vi "Lex Text-Inverted Section-Text.vi"(8 "Error In":errorcluster) -> (0 "Error Out":errorcluster)   [LabVIEW 2018, in "Tests.lvlib" / "Lexer.lvlib"]
uses:
  Lexer.lvlib
  src/Toolkit/Low-Level/Tokens/Text/Text.lvclass
  src/Toolkit/Low-Level/Tokens/InvertedSection/InvertedSection.lvclass
  src/Toolkit/Low-Level/Tokens/Keyable/Keyable.lvclass/Keyable.ctl
  src/Toolkit/Low-Level/Tokens/Keyable/Read Key.vi
  src/Toolkit/Low-Level/Support/Lex String.vi
  <vilib>/Utility/LVClass/Get LV Class Name.vi
  src/Toolkit/Low-Level/Tokens/Contentable/Contentable.lvclass
  src/Toolkit/Low-Level/Tokens/Keyable/Keyable.lvclass
  <vilib>/addons/_JKI Toolkits/Caraya/classes/Test/Test.lvclass
  <vilib>/addons/_JKI Toolkits/Caraya/classes/Assert/Assert.lvclass
  src/Toolkit/Low-Level/Tokens/Abstract/Abstract.lvclass
  Tests.lvlib
  src/Toolkit/Toolkit.lvlib
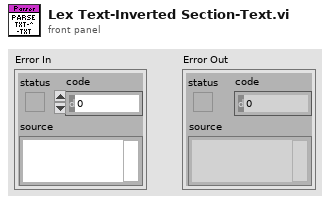
[diagram p1: front panel]
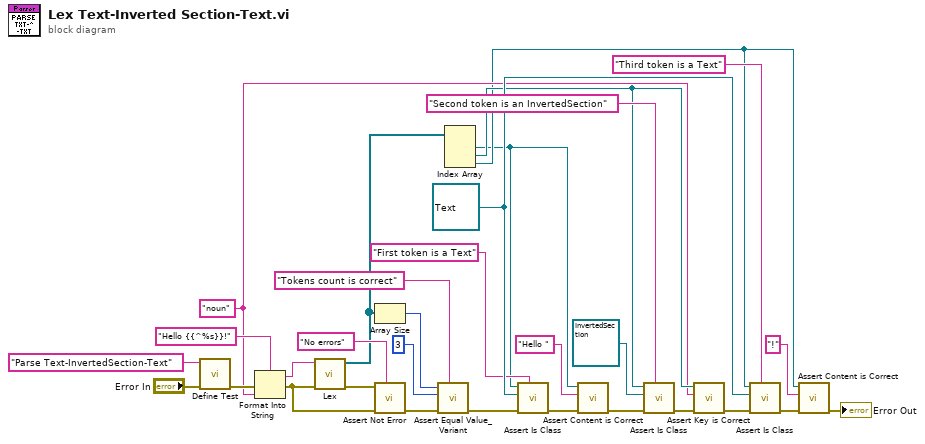
[diagram p0: block diagram]
diagram:
  w15 = refnum<class "Text.lvclass"> refnum ("Mustache.lvlib:Tokens.lvlib:Text.lvclass")
  w9 = "noun" ("String")
  n1 = call <vilib>:"Define Test.vi"("error in (no error)"="Error In", "Label (VI Title)"="Parse Text-InvertedSection-Text") -> ("error out"=w29:errorcluster)  [unwired: 9 in]
  n2 = Format Into String(format string="Hello {{^%s}}!", error in=w29, w9) -> (resulting string=w2:string, error out=w1:errorcluster)  [unwired: 1 in]
  n3 = call-poly "Lex.vi"("Error In"=w1, "Input"=w2) -> ("Error Out"=w3:errorcluster, "Tokens"=w22:refnum<class "Abstract.lvclass">[])  [unwired: 8 in]
  n4 = Array Size(array=w22) -> (size(s)=w25:i32)
  n5 = call <vilib>:"Assert Not Error.vi"("Label"="No errors", "error in (no error)"=w1, "Not Error?"=w3) -> ("error out"=w27:errorcluster)  [unwired: 8 in]
  n6 = call <vilib>:"Assert Equal Value_Variant.vi"("Label"="Tokens count is correct", "error in (no error)"=w27, "Y"=3 ("size(s)"), "X"=w25) -> ("error out"=w23:errorcluster)  [unwired: 7 in]
  n7 = Index Array(array=w22) -> (element #1=w5:refnum<class "Abstract.lvclass">, element #2=w11:refnum<class "Abstract.lvclass">, element #3=w7:refnum<class "Abstract.lvclass">)  [unwired: 3 in]
  n8 = call "Assert Is Class.vi"("Label"="First token is a Text", "Error In"=w23, "Expected"=w15, "Actual"=w5) -> ("Error Out"=w20:errorcluster)  [unwired: 7 in]
  n9 = call "Assert Content is Correct.vi"("Error In"=w20, "Expected"="Hello ", "Token"=w5) -> ("Error Out"=w19:errorcluster)  [unwired: 8 in]
  n10 = call "Assert Is Class.vi"("Label"="Second token is an InvertedSection", "Error In"=w19, "Expected"=refnum<class "InvertedSection.lvclass"> refnum ("Mustache.lvlib:Tokens.lvlib:InvertedSection.lvclass"), "Actual"=w11) -> ("Error Out"=w10:errorcluster)  [unwired: 7 in]
  n11 = call "Assert Key is Correct.vi"("Error In"=w10, "Expected"=w9, "Token"=w11) -> ("Error Out"=w18:errorcluster)  [unwired: 8 in]
  n12 = call "Assert Is Class.vi"("Label"="Third token is a Text", "Error In"=w18, "Expected"=w15, "Actual"=w7) -> ("Error Out"=w17:errorcluster)  [unwired: 7 in]
  n13 = call "Assert Content is Correct.vi"("Error In"=w17, "Expected"="!", "Token"=w7) -> ("Error Out"=→"Error Out":errorcluster)  [unwired: 8 in]
